vi "G4BaseTemplate_Simple_5x6x5_GetProperty.vi"(0 "reference in":refnum<class "G4BaseTemplate_Simple_5x6x5.lvclass">, 11 "Error In":errorcluster) -> (4 "reference out":refnum<class "G4BaseTemplate_Simple_5x6x5.lvclass">, 8 "property":dbl, 15 "Error Out":errorcluster)   [LabVIEW 2020]
uses:
  <resource>/Framework/Providers/Open_GDS/ClassProviders/Provider_EndevoGOOP400/Templates/G4BaseTemplate_Simple_5x6x5/G4BaseTemplate_Simple_5x6x5.lvclass
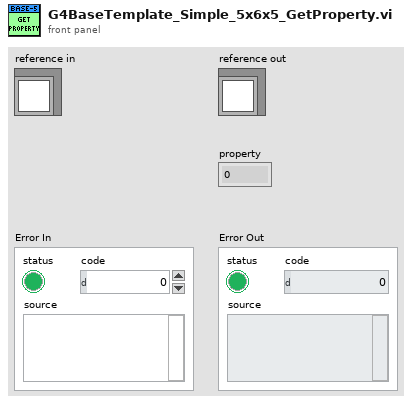
[diagram p1: front panel]
types:
  T1 = typedef "G4BaseTemplate_Simple_5x6x5.lvclass/ObjectAttributes.ctl" = cluster{"Attribute1":dbl}
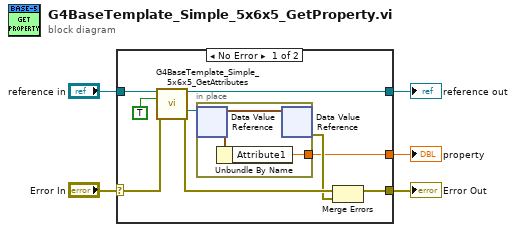
[diagram p0: block diagram]
diagram:
  n1 = case shown="No Error" "Error In" {
    selector: "Error In" -> [w14 w18]
    tunnel: [w12 w18] -> w4
    tunnel: [w9 w17] -> w2
    tunnel: "reference in" -> [w10 w17]
    tunnel: [w8 _] -> w1
    frame No Error {
      n2 = call <resource>:"G4BaseTemplate_Simple_5x6x5_GetAttributes.vi"("reference in"=w10, "OnlyGetDvrReference(False)"=TRUE, "error in (no error)"=w14) -> ("reference out"=w9:refnum<class "G4BaseTemplate_Simple_5x6x5.lvclass">, "DataRef"=w6:refnum<data-value>, "error out"=w13:errorcluster)  [unwired: 9 in, 1 out]
      n3 = in-place {
        in-place-border: [w16] -> w8
        n4 = in-place-dvr #1(w6) -> (w15:T1)  [unwired: 1 out]
        n5 = Unbundle By Name(w15) -> ("Attribute1"=w16:dbl)
        n6 = in-place-dvr #1(w15) -> (w11:errorcluster)  [unwired: 1 out]
      }
      n7 = Merge Errors(w13, w11) -> (w12:errorcluster)
    }
    frame Error {
    }
  }
  "Error Out" <- w4
  "reference out" <- w2
  "property" <- w1
